vi "FGV - Attocube Targets.vi"(4 "error in":errorcluster, 6 "Function":enum16{"write", "read"}(ring), 7 "Targets In":T1) -> (0 "error out":errorcluster, 3 "Targets Out":T1)   [LabVIEW 2016]
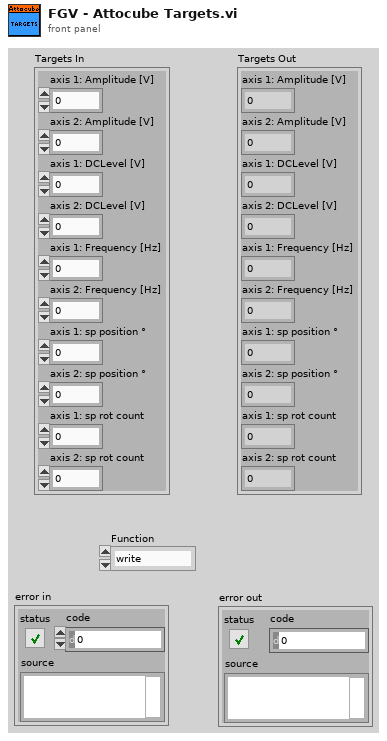
[diagram p1: front panel]
types:
  T1 = cluster{"axis 1: Amplitude [V]":dbl, "axis 2: Amplitude [V]":dbl, "axis 1: DCLevel [V]":dbl, "axis 2: DCLevel [V]":dbl, "axis 1: Frequency [Hz]":dbl, "axis 2: Frequency [Hz]":dbl, "axis 1: sp position °":dbl, "axis 2: sp position °":dbl, "axis 1: sp rot count":dbl, "axis 2: sp rot count":dbl}
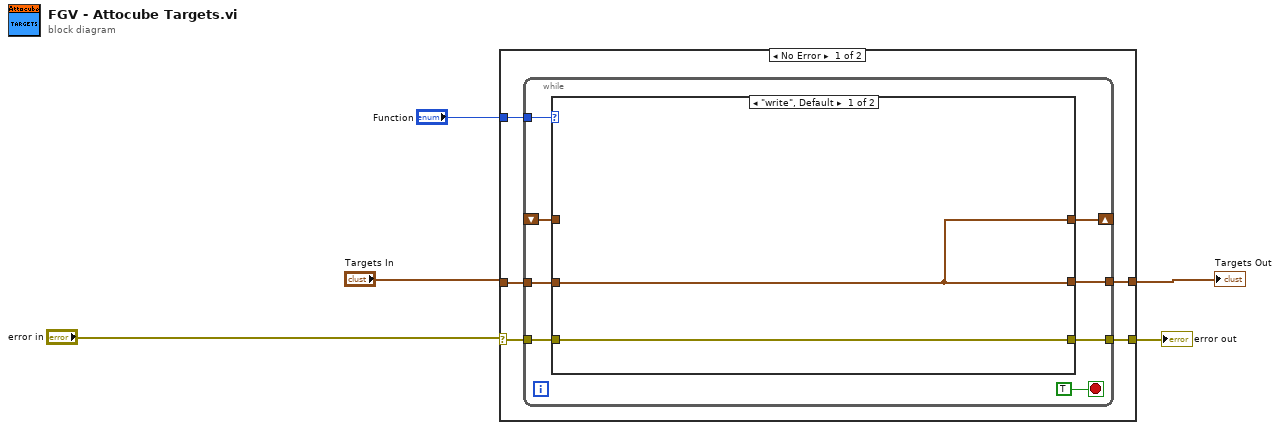
[diagram p0: block diagram]
diagram:
  n1 = case shown="No Error" "error in" {
    selector: "error in" -> [w10 w24]
    tunnel: [w6 w24] -> w5
    tunnel: [w9 w23] -> w2
    tunnel: "Function" -> [w8 _]
    tunnel: "Targets In" -> [w7 w23]
    frame No Error {
      n2 = while {
        shift-right: [w14] -> _
        shift-left: _ -> [w13]
        tunnel: w10 -> [w17]
        tunnel: [w16] -> w9
        tunnel: w8 -> [w15]
        tunnel: w7 -> [w12]
        tunnel: [w11] -> w6
        stop <- TRUE stop-if-true
        n3 = case shown="\"write\", Default" w15 {
          tunnel: w17 -> [w19 w21]
          tunnel: [w20 w22] -> w16
          tunnel: [w20 w22] -> w14
          tunnel: w13 -> [_ w22]
          tunnel: w12 -> [w20 _]
          tunnel: [w19 w21] -> w11
          frame "write", Default {
          }
          frame "read" {
          }
        }
      }
    }
    frame Error {
    }
  }
  "error out" <- w5
  "Targets Out" <- w2
